vi "ad continu conf.vi"(0 "dev":i32, 1 "ch_last":i32, 2 "trig_sl":i32, 3 "clk_sl":i32, 5 "ad_os":i32, 7 "ad_range":i32, 9 "ch_first":i32, 11 "error in (no error)":errorcluster caption="错误输入（无错误）", 12 "freq":i32, 13 "trig_pol":i32, 14 "ext_clk_pol":i32) -> (4 "function return":i32, 15 "error out":errorcluster caption="错误输出")   [LabVIEW 2018, in "恒凯采集卡.lvlib"]
doc: "int ad_continu_conf(int dev,int ad_os,int ad_range,int ch_first,int ch_last,int freq,int trig_sl,int trig_pol,int clk_sl,int ext_clk_pol);"
uses:
  Usb_Daq_V52_32.dll
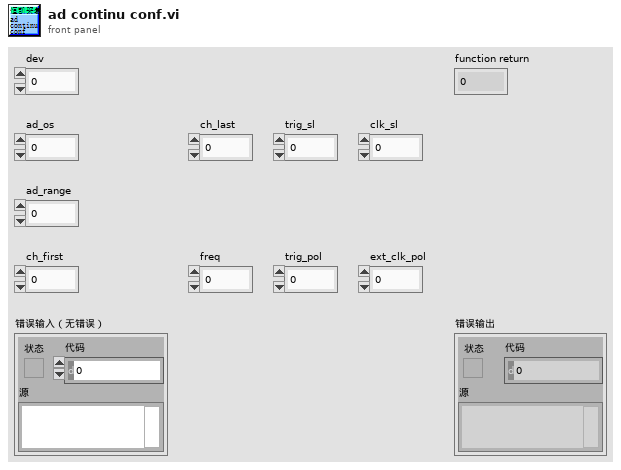
[diagram p1: front panel]
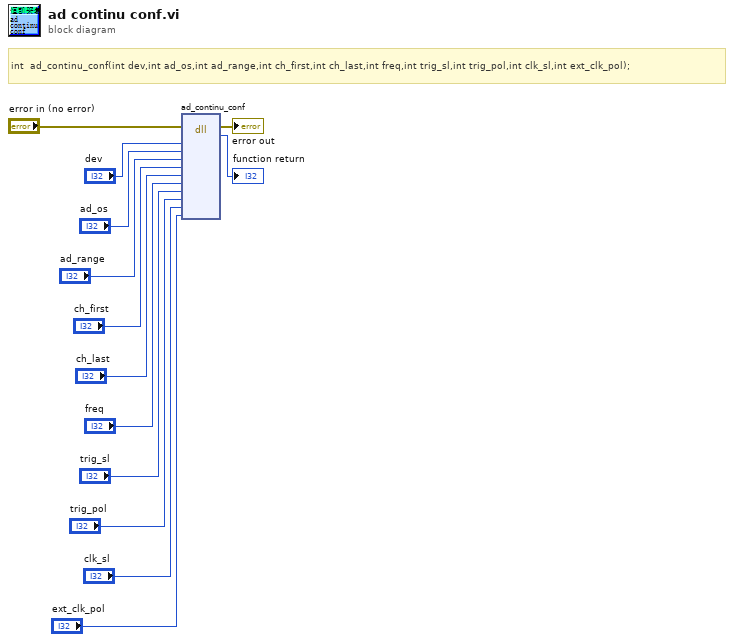
[diagram p0: block diagram]
diagram:
  # "int  ad_continu_conf(int dev,int ad_os,int ad_range,int ch_first,int ch_last,int freq,int trig_sl,int trig_pol,int clk_sl,int ext_clk_pol);"
  n1 = dll-call lib="PTH2Sabs CUsersLenovoDesktop 心肌细胞电信号_231128 -enUsb_Daq_V52_32.*" fn="ad_continu_conf"(error in="error in (no error)", "dev"="dev", "ad_os"="ad_os", "ad_range"="ad_range", "ch_first"="ch_first", "ch_last"="ch_last", "freq"="freq", "trig_sl"="trig_sl", "trig_pol"="trig_pol", "clk_sl"="clk_sl", "ext_clk_pol"="ext_clk_pol") -> (error out=→"error out":errorcluster, →"function return":i32)  [unwired: 12 in, 1 out]
